vi "Group_SetValues.vi"(7 "Data In":dbl[](array[numeric]), 8 "error in (no error)":errorcluster, 10 "Channel Count In":u32, 11 "Group in":refnum<class "Group.lvclass">) -> (0 "error out":errorcluster, 2 "Channel Count Out":u32, 3 "Group out":refnum<class "Group.lvclass">)   [LabVIEW 2023, in "Group.lvclass"]
doc: "Sets the values across this groups channels given a ordered set of double values and a starting index to work with, returning the final index."
uses:
  Group.lvclass
  Group.lvclass/Group.ctl
  Channel/Channel.lvclass
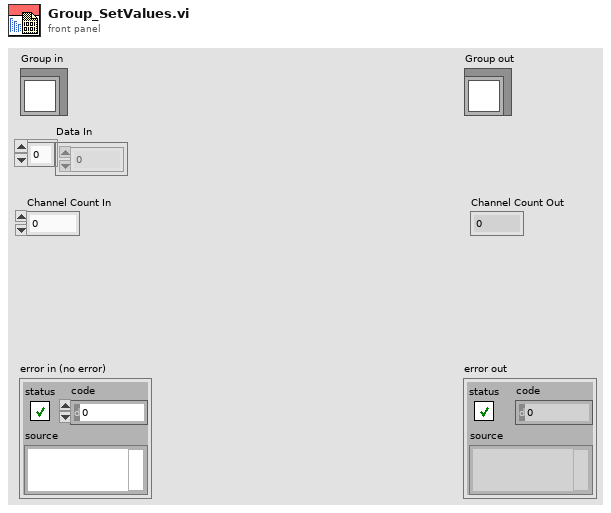
[diagram p1: front panel]
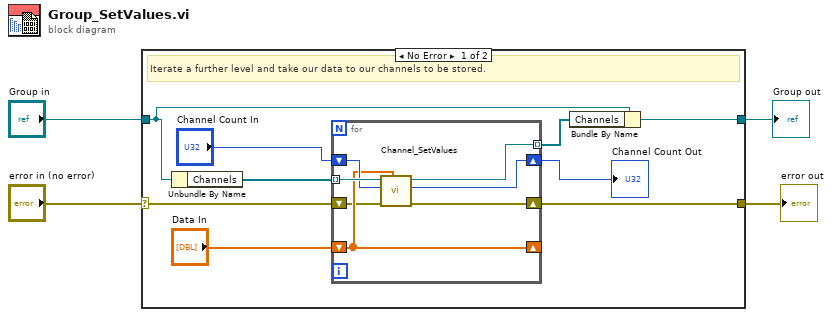
[diagram p0: block diagram]
diagram:
  n1 = case shown="No Error" "error in (no error)" {
    selector: "error in (no error)" -> [w6 w22]
    tunnel: [w5 w22] -> w3
    tunnel: [w8 w21] -> w1
    tunnel: "Group in" -> [w9 w21]
    frame No Error {
      # "Iterate a further level and take our data to our channels to be stored."
      n2 = Unbundle By Name(w9) -> ("Channels"=w13:refnum<class "Channel.lvclass">[])
      n3 = for {
        tunnel: w13 -> [w20] mode=indexing
        shift-right: [w18] -> w11
        shift-left: "Channel Count In" -> [w19]
        shift-right: [w17] -> _
        shift-left: "Data In" -> [w17]
        tunnel: [w16] -> w7 mode=indexing
        shift-right: [w14] -> w5
        shift-left: w6 -> [w15]
        n4 = call-dynamic "Channel_SetValues.vi"("Data In"=w17, "error in (no error)"=w15, "Channel Count"=w19, "Channel in"=w20) -> ("error out"=w14:errorcluster, "Channel Count Out"=w18:u32, "Channel out"=w16:refnum<class "Channel.lvclass">)  [unwired: 5 in]
      }
      "Channel Count Out" <- w11
      n5 = Bundle By Name(cluster=w9, "Channels"=w7) -> (w8:refnum<class "Group.lvclass">)
    }
    frame Error {
    }
  }
  "error out" <- w3
  "Group out" <- w1
